vi "startUp.vi"(8 "error in (no error)":errorcluster, 10 "ScriptEvent":refnum<class "ScriptEvent.lvclass">, 11 "ChangeValueAction in":refnum<class "ChangeValueAction.lvclass">) -> (0 "error out":errorcluster, 3 "ChangeValueAction out":refnum<class "ChangeValueAction.lvclass">)   [LabVIEW 2009, in "Views.lvlib" / "ScriptEditor.lvlib" / "ChangeValueAction.lvclass"]
uses:
  ChangeValueAction.lvclass
  Tools/Scripting/ScriptingEvent/ScriptEvent.lvclass
  ChangeValueAction.lvclass/ChangeValueAction.ctl
  ActionPanel.lvclass
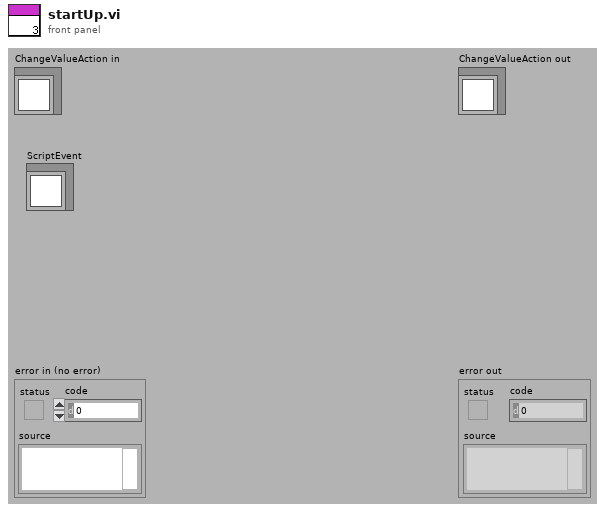
[diagram p1: front panel]
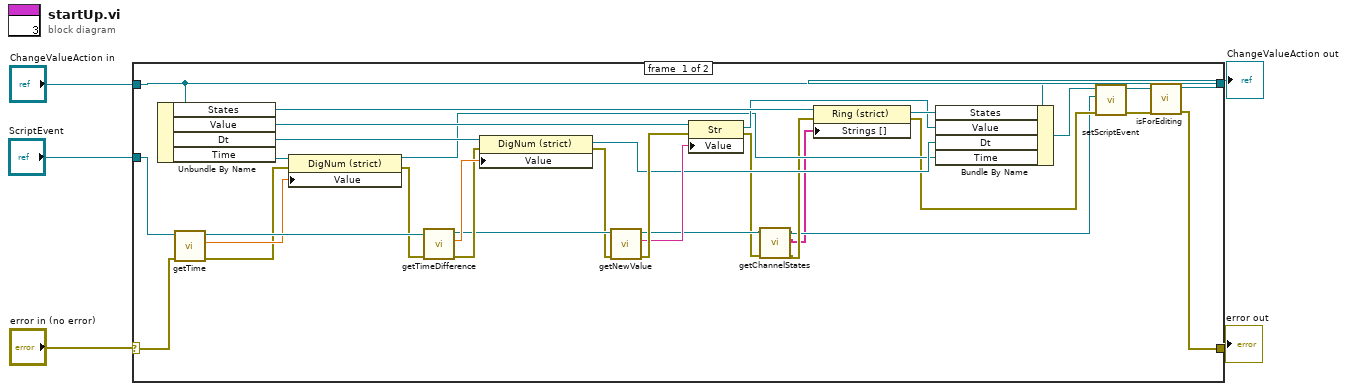
[diagram p0: block diagram]
diagram:
  n1 = case shown="No Error" "error in (no error)" {
    selector: "error in (no error)" -> [w36 w38]
    tunnel: "ChangeValueAction in" -> [w17 w39]
    tunnel: "ScriptEvent" -> [w37 _]
    tunnel: [w8 w39] -> w2
    tunnel: [w6 w38] -> w1
    frame #0 {
      n2 = Unbundle By Name(w17) -> ("States"=w22:refnum<vi>, "Value"=w27:refnum<vi>, "Dt"=w30:refnum<vi>, "Time"=w34:refnum<vi>)
      n3 = call "getTime.vi"("error in (no error)"=w36, "ScriptEvent.lvclass in"=w37) -> ("error out"=w32:errorcluster, "time"=w33:dbl, "ScriptEvent.lvclass out"=w35:refnum<class "ScriptEvent.lvclass">)  [unwired: 7 in]
      n4 = property class="DigNum (strict)"(reference=w34, error in=w32, "Value"=w33) -> (reference out=w18:refnum<vi>, error out=w31:errorcluster)
      n5 = call "getTimeDifference.vi"("error in (no error)"=w31, "ScriptEvent.lvclass in"=w35) -> ("error out"=w28:errorcluster, "time difference"=w29:dbl, "ScriptEvent.lvclass out"=w26:refnum<class "ScriptEvent.lvclass">)  [unwired: 7 in]
      n6 = property class="DigNum (strict)"(reference=w30, error in=w28, "Value"=w29) -> (reference out=w19:refnum<vi>, error out=w25:errorcluster)
      n7 = call "getNewValue.vi"("error in (no error)"=w25, "ScriptEvent.lvclass in"=w26) -> ("error out"=w24:errorcluster, "newValue"=w23:string, "ScriptEvent.lvclass out"=w14:refnum<class "ScriptEvent.lvclass">)  [unwired: 7 in]
      n8 = property class="Str"(reference=w27, error in=w24, "Value"=w23) -> (reference out=w20:refnum<vi>, error out=w13:errorcluster)
      n9 = call-dynamic "getChannelStates.vi"("error in (no error)"=w13, "ScriptEvent in"=w14) -> ("error out"=w12:errorcluster, "statesValues"=w10:string[], "ScriptEvent out"=w11:refnum<class "ScriptEvent.lvclass">)  [unwired: 7 in]
      n10 = property class="Ring (strict)"(reference=w22, error in=w12, "Strings []"=w10) -> (reference out=w21:refnum<vi>, error out=w15:errorcluster)
      n11 = Bundle By Name(cluster=w17, "States"=w21, "Value"=w20, "Dt"=w19, "Time"=w18) -> (w16:refnum<class "ChangeValueAction.lvclass">)
      n12 = call "setScriptEvent.vi"("error in (no error)"=w15, "ScriptEvent.lvclass"=w11, "ActionPanel.lvclass in"=w16) -> ("error out"=w7:errorcluster, "ActionPanel.lvclass out"=w9:refnum<class "ChangeValueAction.lvclass">)  [unwired: 7 in]
      n13 = call-dynamic "isForEditing.vi"("error in (no error)"=w7, "ActionPanel in"=w9) -> ("error out"=w6:errorcluster, "ActionPanel out"=w8:refnum<class "ChangeValueAction.lvclass">)  [unwired: 7 in, 1 out]
    }
    frame #1 {
    }
  }
  "error out" <- w1
  "ChangeValueAction out" <- w2
